vi "Set System References.vi"(8 "error in (no error)":errorcluster) -> (0 "error out":errorcluster, 3 "System Resources":T1)   [LabVIEW 2023]
doc: "This VI gets the system session and system reference and puts it on the appropriate notifier."
uses:
  Type Definitions/System Resources.ctl
  Type Definitions/Payload Class.ctl
  Type Definitions/Enum - Parameters.ctl
  Type Definitions/Device Parameters.ctl
  Type Definitions/Device.ctl
  <vilib>/FPGAPlugInAG/cRIO-9049/niLvFpga_Open_cRIO-9049.vi
  <vilib>/rvi/interface/common/dynamic/niFpgaDynamicAddResources.vi
  <vilib>/FPGAPlugInAG/Dynamic/niLvFpga_Reset_Dynamic.vi
  <vilib>/FPGAPlugInAG/Dynamic/niLvFpga_Run_Dynamic.vi
  <vilib>/rvi/interface/nirviOpenFPGA/nirviOpenFPGA.xnode
  Builds/FPGA Bitfiles/Exec_FPGA.lvbitx
  <vilib>/rvi/interface/nirviMethod/nirviMethod.xnode
  <vilib>/nisyscfg/nisyscfg.lvlib
  <resource>/objmgr/nisysapi.rc
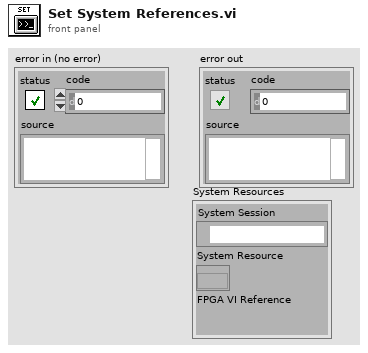
[diagram p1: front panel]
types:
  T1 = typedef "System Resources.ctl" = cluster{"System Session":refnum<k21>, "System Resource":refnum<k20>, "FPGA VI Reference":refnum<k20>}
  T2 = typedef "Device Parameters.ctl" = cluster{"Device":T3}
  T3 = typedef "Device.ctl" = enum32{"None", "Exec", "Aux1", "Aux2", "Aux3"}
  T4 = typedef "Enum - Parameters.ctl" = enum16{"Device Parameters"}
  T5 = typedef "Payload Class.ctl" = enum16{"System State", "Parameters", "Metadata", "Software Monitor", "Data", "Commands"}
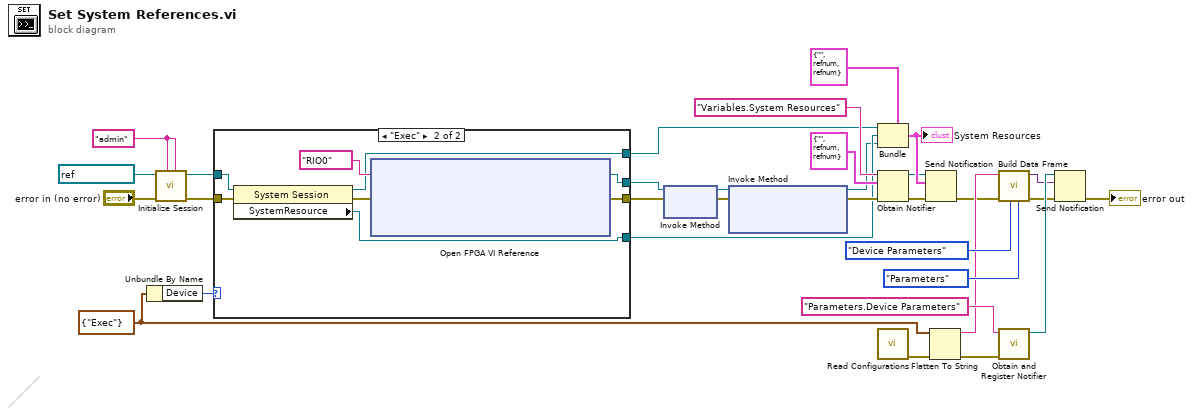
[diagram p0: block diagram]
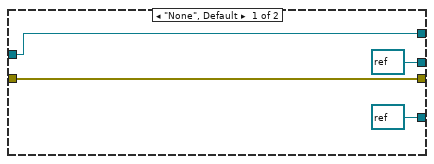
[diagram p2: hidden frame]
diagram:
  w3 = T2 {"Device"=enum."Exec"} ("Device Parameters")
  w23 = "admin" ("User Name")
  n1 = Unbundle By Name(w3) -> ("Device"=w6:T3)
  n2 = call <vilib>:"Initialize Session.vi"("Password"=w23, "User Name"=w23, "error in (no error)"="error in (no error)", "Target (localhost)"=refnum<k21> "localhost") -> ("error out"=w25:errorcluster, "Session out"=w24:refnum<k21>)  [unwired: 6 in]
  n3 = case shown="\"Exec\"" w6 {
    tunnel: w25 -> [w34 w44]
    tunnel: w24 -> [w36 w43]
    tunnel: [w34 w40] -> w20
    tunnel: [refnum<k20> refnum ("FPGA VI Reference Out") w39] -> w4
    tunnel: [w36 w38] -> w17
    tunnel: [refnum<k20> refnum ("SystemResource") w37] -> w16
    frame "None", Default {
    }
    frame "Exec" {
      n4 = property class="System Session"(reference=w43, error in=w44) -> (reference out=w38:refnum<k21>, error out=w42:errorcluster, "SystemResource"=w37:refnum<k20>)
      n5 = xnode "Open FPGA VI Reference"("error in"=w42, "resource name"=tag "RIO0") -> ("FPGA VI Reference Out"=w39:refnum<k20>, "error out"=w40:errorcluster)
    }
  }
  n6 = xnode "Invoke Method"("FPGA VI Reference In"=w4, "error in"=w20) -> ("FPGA VI Reference Out"=w18:refnum<k20>, "error out"=w19:errorcluster)
  n7 = xnode "Invoke Method"("FPGA VI Reference In"=w18, "error in"=w19) -> ("FPGA VI Reference Out"=w2:refnum<k20>, "error out"=w22:errorcluster)  [unwired: 1 in]
  n8 = Bundle(cluster=T1 {"System Session"="", "System Resource"=refnum, "FPGA VI Reference"=refnum} ("System References"), "System Session"=w17, "System Resource"=w16, "FPGA VI Reference"=w2) -> (w30:T1)
  "System Resources" <- w30
  n9 = Obtain Notifier(name (unnamed)="Variables.System Resources", notification data type=T1 {"System Session"="", "System Resource"=refnum, "FPGA VI Reference"=refnum} ("cluster"), error in (no error)=w22) -> (notifier out=w29:refnum<notifier>, error out=w32:errorcluster)  [unwired: 1 in, 1 out]
  n10 = call "Read Configurations.vi"() -> ("error out"=w9:errorcluster)  [unwired: 10 in, 1 out]
  n11 = Send Notification(notification=w30, notifier=w29, error in (no error)=w32) -> (error out=w5:errorcluster)  [unwired: 1 out]
  n12 = Flatten To String(anything=w3, error in (no error)=w9) -> (data string=w11:string, error out=w7:errorcluster)  [unwired: 2 in, 1 out]
  n13 = call "Build Data Frame.vi"("Payload Class (Data)"=Payload_Class."Parameters", "Payload ID (0)"=Enum_-_Parameters."Device Parameters" ("Parameters"), "error in (no error)"=w5, "Payload (Empty String)"=w11) -> ("error out"=w8:errorcluster, "Frame"=w10:variant)  [unwired: 6 in]
  n14 = call "Obtain and Register Notifier.vi"("error in (no error)"=w7, "name (unnamed)"="Parameters.Device Parameters") -> ("notifier out"=w14:refnum<notifier>)  [unwired: 7 in, 2 out]
  n15 = Send Notification(notification=w10, notifier=w14, error in (no error)=w8) -> (error out=→"error out":errorcluster)  [unwired: 1 out]
